vi "Read Multiple.vi"(5 "channel list":string="BL_SEL_0", 6 "current limit range (A)":dbl=3.2e-05 format="%#_6p", 7 "aperture time (s)":dbl=0.0005 format="%#_6p", 8 "error in (no error)":errorcluster, 9 "settling time (s)":dbl=0.0015 format="%#_6p", 10 "voltage level (V)":dbl=0.2 format="%#_6p", 11 "instrument handle":refnum<k15>="PXI1Slot2 (5)") -> (0 "error out":errorcluster, 1 "currents (A)":dbl[][](array[numeric]), 2 "resistances (ohm)":dbl[][](array[numeric]), 3 "instrument handle out":refnum<k15>="PXI1Slot2 (5)")   [LabVIEW 2018]
uses:
  <instrlib>/niDigital/niDigital.llb/niDigital Selected Function.ctl
  <instrlib>/niDigital/niDigital.llb/niDigital Burst Pattern (Burst Only).vi
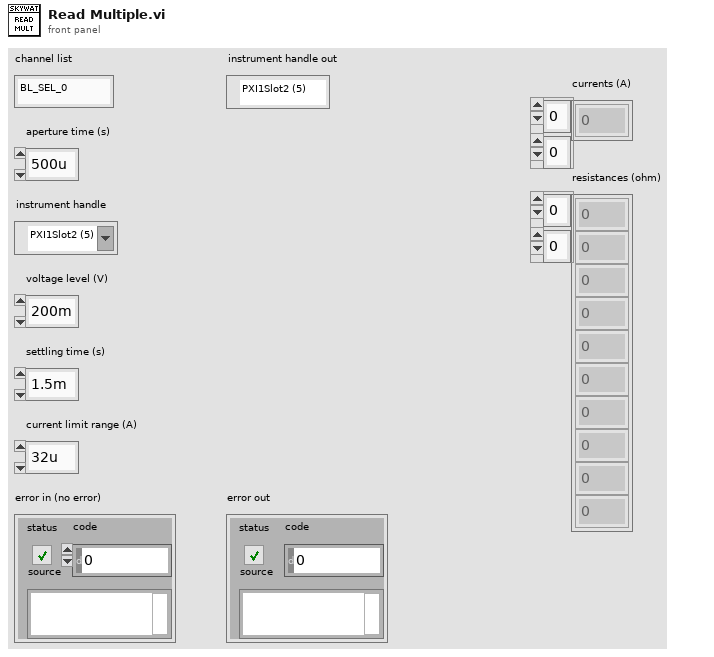
[diagram p1: front panel]
types:
  T1 = typedef "niDigital Selected Function.ctl" = i32
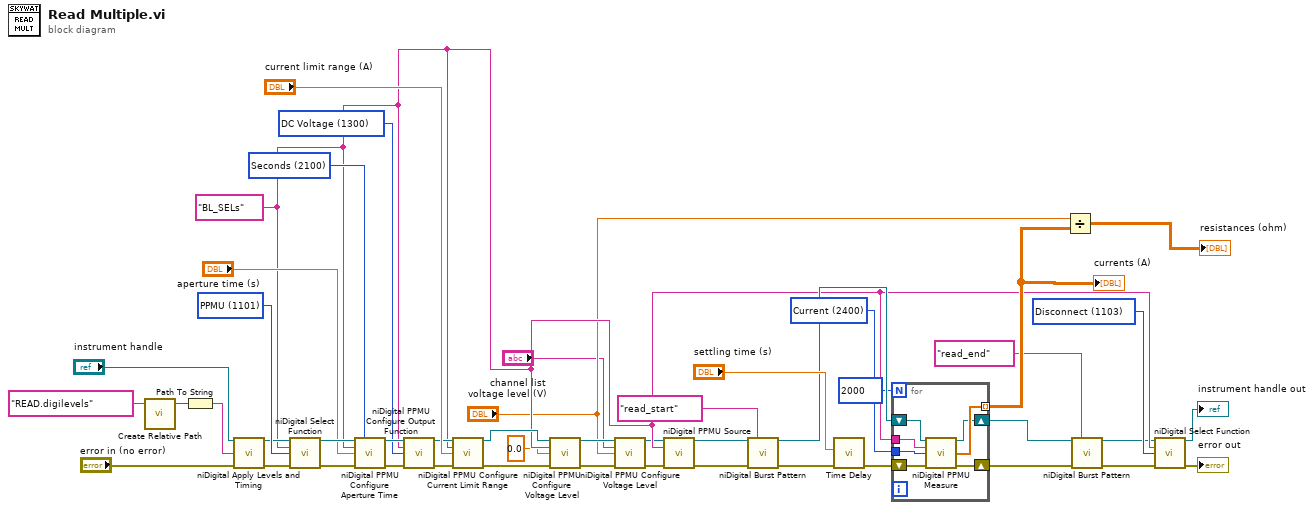
[diagram p0: block diagram]
diagram:
  w15 = "BL_SELs" ("channel list")
  w22 = T1 1103 items=["Digital"=1100, "PPMU"=1101, "Off"=1102, "Disconnect"=1103] ("function")
  w25 = u16 2400 items=["Voltage"=2401, "Current"=2400] ("measurement type")
  w44 = T1 1101 items=["Digital"=1100, "PPMU"=1101, "Off"=1102, "Disconnect"=1103] ("function")
  w31 = u16 2100 items=["Seconds"=2100] ("aperture time units")
  w35 = u16 1300 items=["DC Voltage"=1300, "DC Current"=1301] ("output function")
  n1 = call "Create Relative Path.vi"("file name"="READ.digilevels" ("levels sheet")) -> ("appended path"=w28:path)  [unwired: 4 in]
  n2 = Path To String(path=w28) -> (string=w26:string)
  n3 = call <instrlib>:"niDigital Apply Levels and Timing.vi"("instrument handle"="instrument handle", "levels sheet"=w26, "error in"="error in (no error)") -> ("instrument handle out"=w21:refnum<k15>, "error out"=w20:errorcluster)  [unwired: 11 in]
  n4 = call <instrlib>:"niDigital Select Function.vi"("instrument handle"=w21, "channel list"=w15, "function"=w44, "error in"=w20) -> ("instrument handle out"=w42:refnum<k15>, "error out"=w43:errorcluster)  [unwired: 10 in]
  n5 = call <instrlib>:"niDigital PPMU Configure Aperture Time.vi"("instrument handle"=w42, "aperture time units"=w31, "channel list"=w15, "aperture time"="aperture time (s)", "error in"=w43) -> ("instrument handle out"=w38:refnum<k15>, "error out"=w39:errorcluster)  [unwired: 9 in]
  n6 = call <instrlib>:"niDigital PPMU Configure Output Function.vi"("instrument handle"=w38, "channel list"=w15, "output function"=w35, "error in"=w39) -> ("instrument handle out"=w33:refnum<k15>, "error out"=w36:errorcluster)  [unwired: 10 in]
  n7 = call <instrlib>:"niDigital PPMU Configure Current Limit Range.vi"("instrument handle"=w33, "channel list"=w15, "current limit range (A)"="current limit range (A)", "error in"=w36) -> ("instrument handle out"=w34:refnum<k15>, "error out"=w37:errorcluster)  [unwired: 10 in]
  n8 = call <instrlib>:"niDigital PPMU Configure Voltage Level.vi"("instrument handle"=w34, "channel list"=w15, "voltage level (V)"=0.0, "error in"=w37) -> ("instrument handle out"=w14:refnum<k15>, "error out"=w11:errorcluster)  [unwired: 10 in]
  n9 = call <instrlib>:"niDigital PPMU Configure Voltage Level.vi"("instrument handle"=w14, "channel list"="channel list", "voltage level (V)"="voltage level (V)", "error in"=w11) -> ("instrument handle out"=w13:refnum<k15>, "error out"=w12:errorcluster)  [unwired: 10 in]
  n10 = call <instrlib>:"niDigital PPMU Source.vi"("instrument handle"=w13, "channel list"=w15, "error in"=w12) -> ("instrument handle out"=w19:refnum<k15>, "error out"=w18:errorcluster)  [unwired: 11 in]
  n11 = call-poly <instrlib>:"niDigital Burst Pattern.vi"("instrument handle"=w19, "start label"="read_start", "error in"=w18) -> ("instrument handle out"=w16:refnum<k15>, "error out"=w17:errorcluster)  [unwired: 11 in]
  n12 = call "Time Delay"("error in (no error)"=w17, "Delay Time (s)"="settling time (s)") -> ("error out"=w47:errorcluster)  [unwired: 9 in]
  n13 = for {
    N: 2000 -> [_]
    tunnel: [w53] -> w46 mode=indexing
    tunnel: w25 -> [w52]
    tunnel: w15 -> [w50]
    shift-right: [w48] -> w6
    shift-left: w47 -> [w54]
    shift-right: [w49] -> w7
    shift-left: w16 -> [w51]
    n14 = call <instrlib>:"niDigital PPMU Measure.vi"("instrument handle"=w51, "channel list"=w50, "measurement type"=w52, "error in"=w54) -> ("instrument handle out"=w49:refnum<k15>, "measurements"=w53:dbl[], "error out"=w48:errorcluster)  [unwired: 9 in]
  }
  "currents (A)" <- w46
  n15 = Divide(x="voltage level (V)", y=w46) -> (x/y=→"resistances (ohm)":dbl[][])
  n16 = call-poly <instrlib>:"niDigital Burst Pattern.vi"("instrument handle"=w7, "start label"="read_end", "error in"=w6) -> ("instrument handle out"=w3:refnum<k15>, "error out"=w2:errorcluster)  [unwired: 11 in]
  n17 = call <instrlib>:"niDigital Select Function.vi"("instrument handle"=w3, "channel list"=w15, "function"=w22, "error in"=w2) -> ("instrument handle out"=→"instrument handle out":refnum<k15>, "error out"=→"error out":errorcluster)  [unwired: 10 in]
